vi "Solution part 2b.vi"(11 "data?":bool) -> ()   [LabVIEW 2020]
panel:
  out "final loop index":u64
  out "loop index":u64
  out "max bus ID":cluster{"bus id":i32, "index":i32}
  in  "manual input":string
  in  "file input?":bool
  out "Timestamp":u64
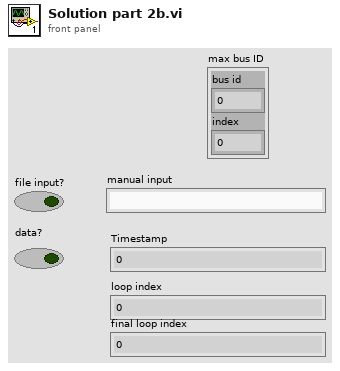
[diagram p1: front panel]
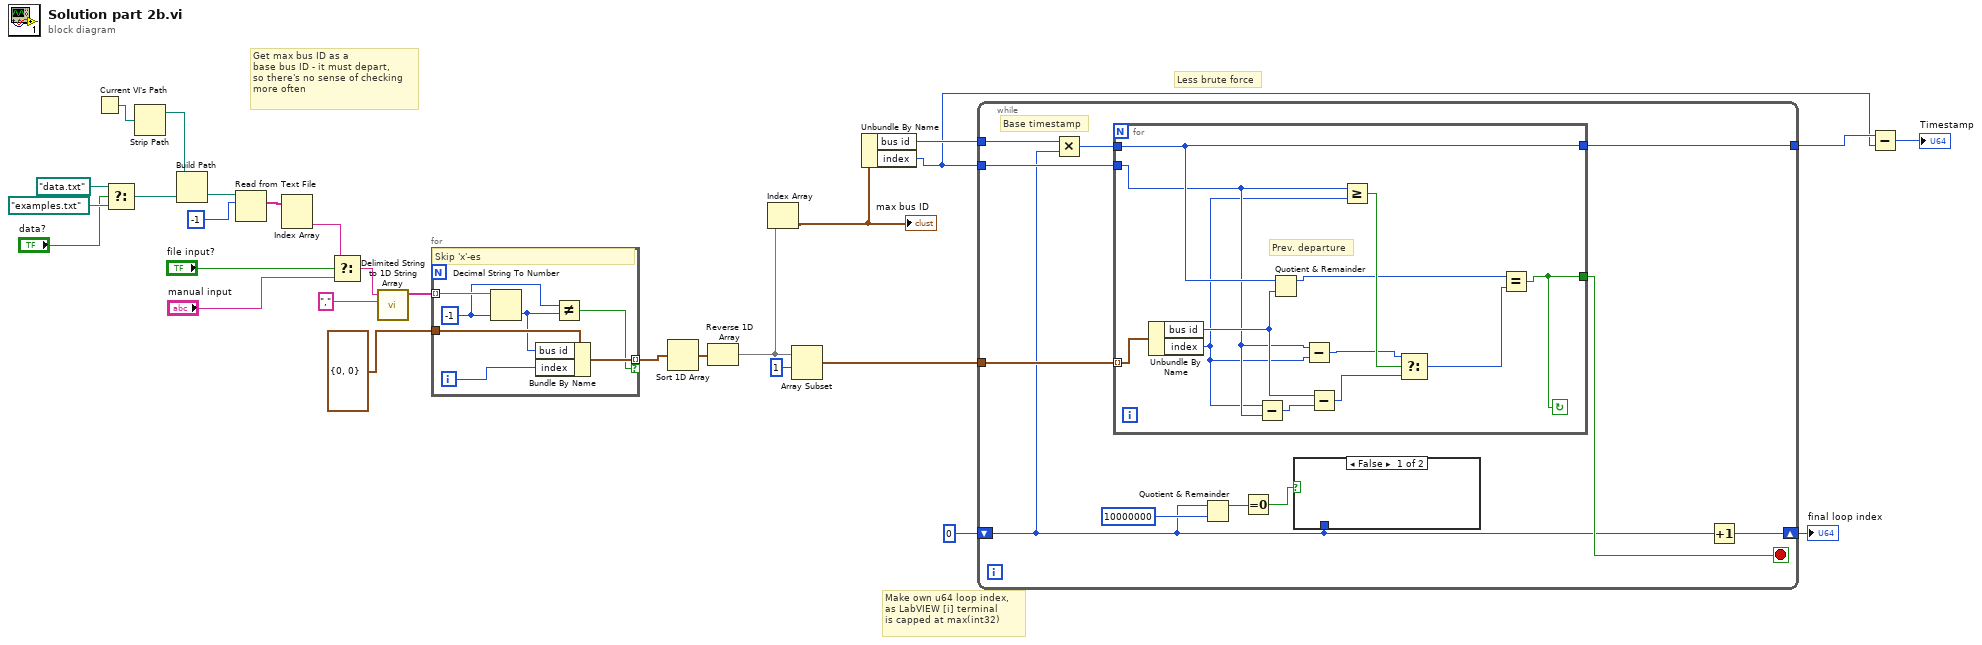
[diagram p0: block diagram]
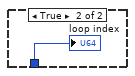
[diagram p2: hidden frame]
diagram:
  # "Less brute force"
  # "Make own u64 loop index,\nas LabVIEW [i] terminal\nis capped at max(int32)"
  # "Get max bus ID as a\nbase bus ID - it must depart,\nso there's no sense of checking\nmore often"
  n1 = Current VI's Path() -> (path=w25:path)
  n2 = Select(t=path "data.txt", s="data?", f=path "examples.txt") -> (s? t:f=w26:path)
  n3 = Strip Path(path=w25) -> (stripped path=w24:path)  [unwired: 1 out]
  n4 = Build Path(base path=w24, name or relative path=w26) -> (appended path=w23:path)
  n5 = Read from Text File(file (use dialog)=w23, count=-1) -> (text=w20:string[])  [unwired: 2 in, 3 out]
  n6 = Index Array(array=w20) -> (element #2=w19:string)  [unwired: 2 in, 1 out]
  n7 = Select(t=w19, s="file input?", f="manual input") -> (s? t:f=w17:string)
  n8 = call <vilib>:"Delimited String to 1D String Array.vi"("delimiter"=",", "delimited string"=w17) -> ("string array"=w14:string[])  [unwired: 9 in]
  n9 = for {
    tunnel: w14 -> [w35] mode=indexing
    tunnel: cluster{"bus id":i32, "index":i32} {"bus id"=0, "index"=0} -> [w34]
    tunnel: [w32] -> w5 mode=indexing if=w29
    i -> [w33]
    w30 = -1 ("default (0 I32)")
    # "Skip 'x'-es"
    n10 = Decimal String To Number(string=w35, default (0L)=w30) -> (number=w31:i32)  [unwired: 1 in, 1 out]
    n11 = Bundle By Name(cluster=w34, "bus id"=w31, "index"=w33) -> (w32:cluster{"bus id":i32, "index":i32})
    n12 = Not Equal?(x=w30, y=w31) -> (x != y?=w29:bool)
  }
  n13 = Sort 1D Array(array=w5) -> (sorted array=w10:cluster{"bus id":i32, "index":i32}[])
  n14 = Reverse 1D Array(array=w10) -> (reversed array=w8:cluster{"bus id":i32, "index":i32}[])
  n15 = Index Array(array=w8) -> (element=w9:cluster{"bus id":i32, "index":i32})  [unwired: 1 in]
  "max bus ID" <- w9
  n16 = Array Subset(array=w8, index=1) -> (w6:cluster{"bus id":i32, "index":i32}[])  [unwired: 1 in]
  n17 = Unbundle By Name(w9) -> ("bus id"=w11:i32, "index"=w3:i32)
  n18 = while {
    tunnel: w11 -> [w45]
    shift-right: [w46] -> w1
    shift-left: u64 0 ("index") -> [w36]
    tunnel: w6 -> [w42]
    tunnel: w3 -> [w41]
    tunnel: [w40] -> w4
    stop <- w43 stop-if-true
    # "Base timestamp"
    n19 = Multiply(x=w45, y=w36) -> (x*y=w44:u64)
    n20 = for {
      tunnel: [w59] -> w43
      tunnel: w44 -> [w55]
      tunnel: w42 -> [w58] mode=indexing
      tunnel: w41 -> [w49]
      tunnel: [w55] -> w40
      stop <- w59 continue-if-true
      # "Prev. departure"
      n21 = Unbundle By Name(w58) -> ("bus id"=w53:i32, "index"=w48:i32)
      n22 = Subtract(x=w48, y=w49) -> (x-y=w52:i32)
      n23 = Quotient & Remainder(x=w55, y=w53) -> (x-y*floor(x/y)=w54:u64)  [unwired: 1 out]
      n24 = Subtract(x=w49, y=w48) -> (x-y=w51:i32)
      n25 = Subtract(x=w53, y=w52) -> (x-y=w50:i32)
      n26 = Greater Or Equal?(x=w49, y=w48) -> (x >= y?=w57:bool)
      n27 = Select(t=w51, s=w57, f=w50) -> (s? t:f=w56:i32)
      n28 = Equal?(x=w54, y=w56) -> (x = y?=w59:bool)
    }
    n29 = Quotient & Remainder(x=w36, y=u64 10000000) -> (x-y*floor(x/y)=w38:u64)  [unwired: 1 out]
    n30 = Equal To 0?(x=w38) -> (x = 0?=w37:bool)
    n31 = case shown="False" w37 {
      tunnel: w36 -> [_ w47]
      frame False {
      }
      frame True {
        "loop index" <- w47
      }
    }
    n32 = Increment(x=w36) -> (x+1=w46:u64)
  }
  "final loop index" <- w1
  n33 = Subtract(x=w4, y=w3) -> (x-y=→"Timestamp":u64)
